vi "Command Drive Cube.vi"(7 "Startup":bool, 9 "Timeout":u32, 11 "Speed":dbl) -> (2 "Right Wheel":dbl, 3 "Left Wheel":dbl, 4 "Reinit":bool, 6 "Completed":bool)   [LabVIEW 2017]
uses:
  Intake/Intake Globals.vi
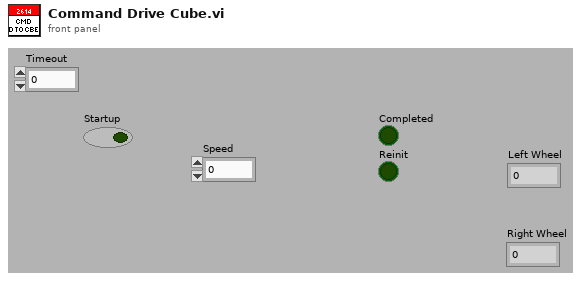
[diagram p1: front panel]
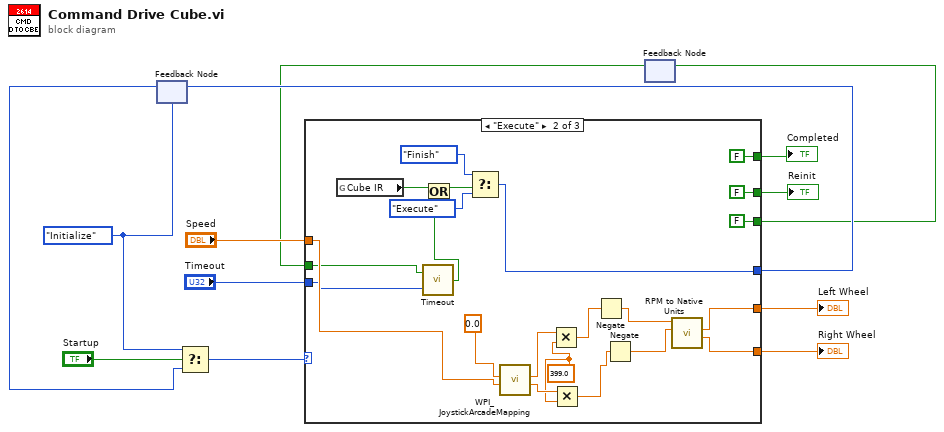
[diagram p0: block diagram]
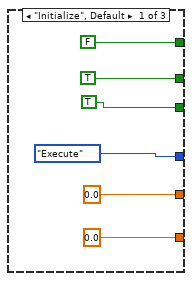
[diagram p2: hidden frame]
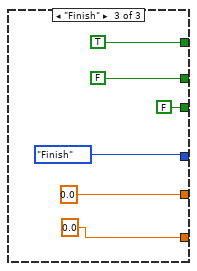
[diagram p3: hidden frame]
diagram:
  w11 = enum16{"Initialize", "Execute", "Finish"}."Initialize"
  n1 = feedback #1(w11) -> (w7:enum16{"Initialize", "Execute", "Finish"})
  n2 = Select(t=w11, s="Startup", f=w7) -> (s? t:f=w12:enum16{"Initialize", "Execute", "Finish"})
  n3 = feedback #2() -> (w1:bool)  [unwired: 1 in]
  n4 = case shown="\"Execute\"" w12 {
    tunnel: [FALSE FALSE TRUE] -> w10
    tunnel: [TRUE FALSE FALSE] -> w9
    tunnel: [enum16{"Initialize", "Execute", "Finish"}."Execute" w37 enum16{"Initialize", "Execute", "Finish"}."Finish"] -> w8
    tunnel: "Speed" -> [_ w35 _]
    tunnel: [0.0 ("Left Wheel Velocity") w26 0.0] -> w5
    tunnel: [0.0 ("Right Wheel Velocity") w25 0.0] -> w4
    tunnel: "Timeout" -> [_ w24 _]
    tunnel: [TRUE FALSE FALSE] -> w2
    tunnel: w1 -> [_ w23 _]
    frame "Initialize", Default {
    }
    frame "Execute" {
      w29 = 399.0
      n5 = global read "Intake Globals.vi" "Cube IR"() -> (w36:bool)
      n6 = call "Timeout.vi"("Timeout"=w24, "Initialize"=w23) -> ("Timed Out?"=w21:bool)
      n7 = Or(x=w36, y=w21) -> (x .or. y?=w22:bool)
      n8 = Select(t=enum16{"Initialize", "Execute", "Finish"}."Finish", s=w22, f=enum16{"Initialize", "Execute", "Finish"}."Execute") -> (s? t:f=w37:enum16{"Initialize", "Execute", "Finish"})
      n9 = call <vilib>:"WPI_JoystickArcadeMapping.vi"("Y axis value"=w35, "X axis value"=0.0) -> ("Right Motor Value"=w32:dbl, "Left Motor Value"=w33:dbl)  [unwired: 8 in]
      n10 = Multiply(x=w33, y=w29) -> (x*y=w30:dbl)
      n11 = Multiply(x=w32, y=w29) -> (x*y=w31:dbl)
      n12 = Negate(x=w30) -> (-x=w28:dbl)
      n13 = Negate(x=w31) -> (-x=w27:dbl)
      n14 = call "RPM to Native Units.vi"("Right RPM"=w27, "Left RPM"=w28) -> ("Right Out"=w25:dbl, "Left Out"=w26:dbl)  [unwired: 6 in, 1 out]
    }
    frame "Finish" {
    }
  }
  "Completed" <- w10
  "Reinit" <- w9
  "Left Wheel" <- w5
  "Right Wheel" <- w4
  n15 = feedback-in #1(w8) -> ()
  n16 = feedback-in #2(w2) -> ()
